vi "Reopen VISA.vi"(0 "VISA resource name":refnum<visa-resource-name>, 5 "IP Address Changed (F)?":bool, 7 "IP Address (000.000.000.000)":string="000.000.000.000", 11 "error in (no error)":errorcluster) -> (4 "VISA resource name out":refnum<visa-resource-name>, 15 "error out":errorcluster)   [LabVIEW 2020, in "eec EST 300.lvlib"]
doc: "Reads the response from the instrument, when it is connected in serial mode (This is because the instrument sends the ACK or NACK automatically in this mode of communication)\n\nThis is a Private type VI and meant for getting the acknowledgement alone."
uses:
  <instrlib>/eec EST 300/eec EST 300.lvlib
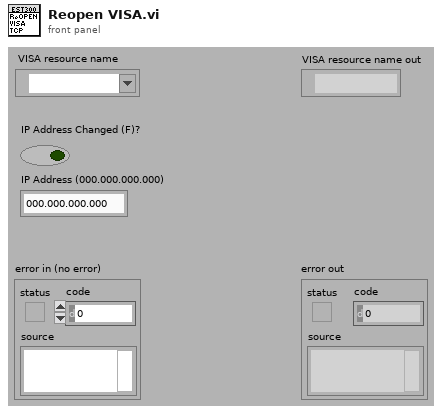
[diagram p1: front panel]
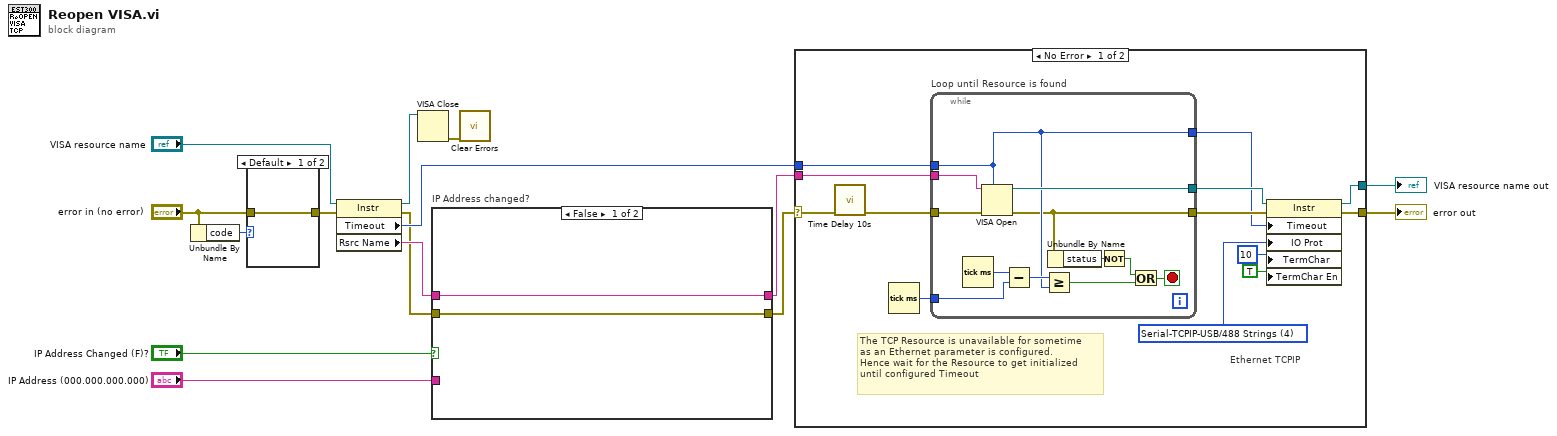
[diagram p0: block diagram]
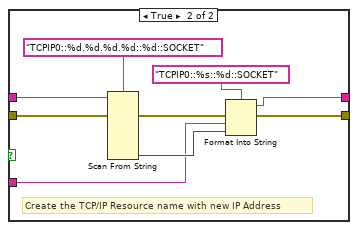
[diagram p2: hidden frame]
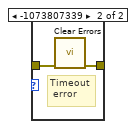
[diagram p3: hidden frame]
diagram:
  n1 = Unbundle By Name("error in (no error)") -> ("code"=w12:i32)
  n2 = case shown="Default" w12 {
    tunnel: "error in (no error)" -> [w16 w18]
    tunnel: [w16 w17] -> w4
    frame Default {
    }
    frame -1073807339 {
      # "Timeout\n error"
      n3 = call <vilib>:"Clear Errors.vi"("error in (no error)"=w18) -> ("error out"=w17:errorcluster)  [unwired: 5 in, 1 out]
    }
  }
  n4 = property on="Property Node" class="Instr"(reference="VISA resource name", error in=w4) -> (reference out=w7:refnum<visa-resource-name>, error out=w3:errorcluster, "Timeout"=w10:u32, "Rsrc Name"=w9:string)
  n5 = VISA Close(VISA resource name=w7) -> (error out=w1:errorcluster)  [unwired: 1 in]
  n6 = case "IP Address changed?" shown="False" "IP Address Changed (F)?" {
    tunnel: w9 -> [w20 w25]
    tunnel: "IP Address (000.000.000.000)" -> [_ w24]
    tunnel: [w20 w23] -> w6
    tunnel: w3 -> [w19 w22]
    tunnel: [w19 w21] -> w2
    frame False {
    }
    frame True {
      # "Create the TCP/IP Resource name with new IP Address"
      n7 = Scan From String(format string="TCPIP0::%d.%d.%d.%d::%d::SOCKET", input string=w25, error in=w22) -> (error out=w29:errorcluster, output 5=w26:i32)  [unwired: 10 in, 2 out]
      n8 = Format Into String(format string="TCPIP0::%s::%d::SOCKET", error in=w29, w24, w26) -> (resulting string=w23:string, error out=w21:errorcluster)  [unwired: 1 in]
    }
  }
  n9 = call <vilib>:"Clear Errors.vi"("error in (no error)"=w1) -> ()  [unwired: 5 in, 2 out]
  n10 = case shown="No Error" w2 {
    selector: w2 -> [w30 w56]
    tunnel: w6 -> [w33 w55]
    tunnel: [w37 w56] -> w15
    tunnel: [w36 w55] -> w14
    tunnel: w10 -> [w32 _]
    frame No Error {
      w40 = u16 4 items=["Normal"=1, "VXI/FDC"=2, "GPIB/HS488"=3, "Serial-TCPIP-USB/488 Strings"=4, "USBTMC/Vendor-Specific"=5] ("Message Based Settings:IO Protocol")
      # "The TCP Resource is unavailable for sometime\nas an Ethernet parameter is configured.\nHence wait for the Resource to get initialized\nuntil configured Timeout"
      # "Ethernet TCPIP"
      n11 = call "Time Delay 10s"("error in (no error)"=w30) -> ("error out"=w31:errorcluster)  [unwired: 10 in]
      n12 = Tick Count (ms)() -> (millisecond timer value=w35:u32)
      n13 = while "Loop until Resource is found" {
        tunnel: [w43] -> w39
        tunnel: [w46] -> w38
        tunnel: w33 -> [w54]
        tunnel: w31 -> [w53]
        tunnel: w35 -> [w51]
        tunnel: [w44] -> w34
        tunnel: w32 -> [w44]
        stop <- w47 stop-if-true
        n14 = Tick Count (ms)() -> (millisecond timer value=w52:u32)
        n15 = VISA Open(timeout (0)=w44, error in (no error)=w53, VISA resource name=w54) -> (VISA resource name=w46:refnum<visa-resource-name>, error out=w43:errorcluster)  [unwired: 2 in]
        n16 = Subtract(x=w52, y=w51) -> (x-y=w45:u32)
        n17 = Greater Or Equal?(x=w45, y=w44) -> (x >= y?=w48:bool)
        n18 = Unbundle By Name(w43) -> ("status"=w50:bool)
        n19 = Not(x=w50) -> (.not. x?=w49:bool)
        n20 = Or(x=w49, y=w48) -> (x .or. y?=w47:bool)
      }
      n21 = property on="Property Node" class="Instr"(reference=w38, error in=w39, "Timeout"=w34, "IO Prot"=w40, "TermChar"=u8 10 ("Message Based Settings:Termination Character"), "TermChar En"=TRUE ("Message Based Settings:Termination Character Enable")) -> (reference out=w36:refnum<visa-resource-name>, error out=w37:errorcluster)
    }
    frame Error {
    }
  }
  "VISA resource name out" <- w14
  "error out" <- w15
